vi "通信并与其他模块交互 (子VI).vi"() -> ()   [LabVIEW 2016, in "质控单元.lvlib"]
uses:
  <vilib>/Plasmionique/MB Master/MB_Master_TCP/MB_Master_TCP.lvclass
  D:/Program Files (x86)/National Instruments/LabVIEW 2016/vi.lib/Plasmionique/MB Master/MB_Master/MB_Master.lvclass
  <vilib>/Plasmionique/MB Master/MB_Master/MB_Master.lvclass
  <vilib>/Plasmionique/MB Master/MB Master.lvlib
  <vilib>/Utility/config.llb/NI_LVConfig.lvlib
panel:
  out "CODCr测量状态":u16[](array[numeric])
  out "CODMn测量状态":u16[](array[numeric])
  out "总氮测量状态":u16[](array[numeric])
  out "总磷测量状态":u16[](array[numeric])
  out "氨氮测量状态":u16[](array[numeric])
  out "通讯状态":bool
  out "待处理插入数量":i32
  out "元素":cluster{"命令":string}[](array[cluster])
  out "队列中元素数量":i32
  in  "starting address 6":u16
  in  "values 6":u16[](array[numeric])
  in  "starting address 5":u16
  in  "values 5":u16[](array[numeric])
  in  "starting address 4":u16
  in  "values 4":u16[](array[numeric])
  in  "starting address 3":u16
  in  "values 3":u16[](array[numeric])
  in  "starting address 2":u16
  in  "values 2":u16[](array[numeric])
  in  "values":u16[](array[numeric])
  in  "starting address":u16
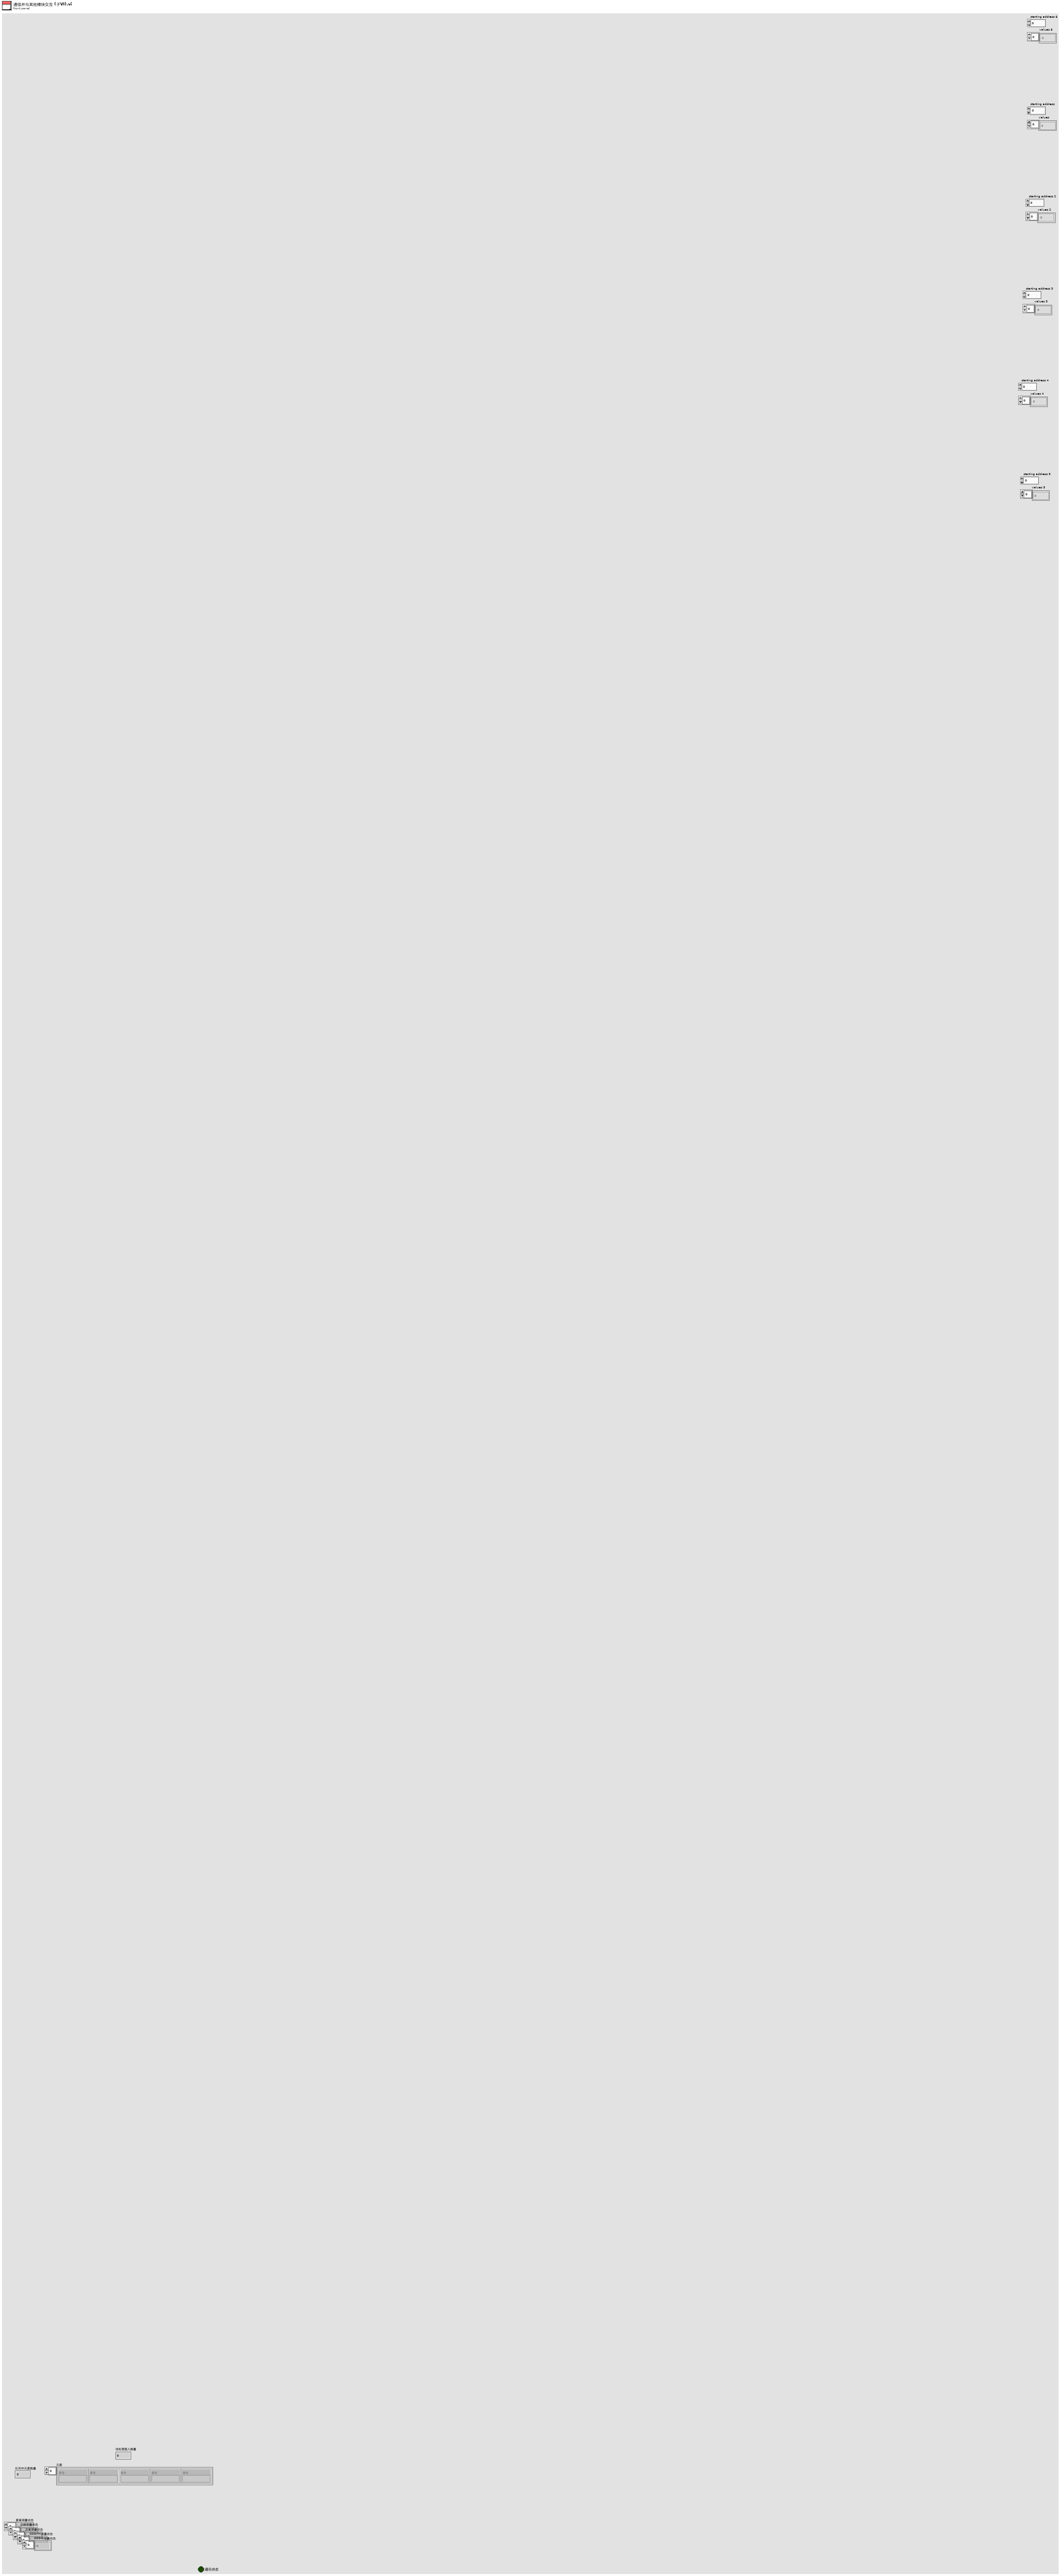
[diagram p1: front panel]
types:
  T1 = typedef "NI_LVConfig.lvlib/Config Data RefNum.ctl" = refnum<k1>
  T2 = cluster{"因子编码":u32, "单位":u16, "标样参考值":sgl, "水样数据时间":timestamp, "水样实测值":sgl, "水样数据标识":string, "标样数据时间":timestamp, "标样实测值":sgl, "标样数据标识":string, "空白数据时间":timestamp, "空白实测值":sgl, "空白数据标识":string, "零点核查数据时间":timestamp, "零点核查实测值":sgl, "零点核查数据标识":string, "跨度核查数据时间":timestamp, "跨度核查实测值":sgl, "跨度核查数据标识":string, "加标回收数据时间":timestamp, "加标回收实测值":sgl, "加标回收数据标识":string, "平行样数据时间":timestamp, "平行样实测值":sgl, "平行样数据标识":string}
  T3 = cluster{"系统时间":timestamp, "工作状态":enum16{"空闲", "水样测试", "标样核查", "零点核查", "跨度核查", "空白测试", "平行样测试", "加标回收", "空白校准", "标样校准", "初始化（清洗）"}, "测量模式":enum16{"待机", "连续模式", "周期模式", "定点模式", "受控模式", "手动模式"}, "告警代码":enum16{"无告警", "缺试剂告警", "缺水样告警", "缺蒸馏水告警", "缺标液告警", "仪表漏液告警", "标定异常告警", "超量程告警", "加热异常", "低试剂预警", "超上限告警", "超下限告警", "仪表内部其他异常", "滴定异常告警", "电极异常告警", "量程切换告警", "参数设置告警", "PH电极电位异常", "电导率电极异常", "浊度光度异常", "溶解氧电极异常", "溶解氧光强异常", "温度异常告警", "PH异常告警", "溶解氧异常告警", "电导率异常告警", "浊度异常告警", "叶绿素异常告警", "藻密度异常告警", "蓝绿藻异常告警", "ORP异常告警", "氨氮异常告警", "清洁刷异常告警", "SD卡异常告警", "蓝牙异常告警", "Wifi异常告警", "流程异常告警"}, "故障代码":enum16{"无故障", "电机故障", "温度故障", "通讯故障", "滴定故障"}, "日志代码":u16, "软件版本":u16, "F0":sgl, "F1":sgl, "F2":sgl, "F3":sgl, "T":sgl, "H":sgl, "id":u16, "flowid":u16, "量程":u16, "总磷控温温度1":sgl, "营养盐控温温度2":sgl, "ADC":sgl}
  T4 = cluster{"Registers[0]":u16, "Registers[1]":u16, "Registers[2]":u16, "Registers[3]":u16, "Registers[4]":u16, "Registers[5]":u16, "Registers[6]":u16, "Registers[7]":u16, "Registers[8]":u16, "Registers[9]":u16, "Registers[10]":u16, "Registers[11]":u16, "Registers[12]":u16, "Registers[13]":u16, "Registers[14]":u16, "Registers[15]":u16, "Registers[16]":u16, "Registers[17]":u16, "Registers[18]":u16, "Registers[19]":u16, "Registers[20]":u16, "Registers[21]":u16, "Registers[22]":u16, "Registers[23]":u16, "Registers[24]":u16, "Registers[25]":u16, "Registers[26]":u16, "Registers[27]":u16, "Registers[28]":u16, "Registers[29]":u16, "Registers[30]":u16, "Registers[31]":u16, "Registers[32]":u16, "Registers[33]":u16, "Registers[34]":u16, "Registers[35]":u16, "Registers[36]":u16, "Registers[37]":u16, "Registers[38]":u16, "Registers[39]":u16, "Registers[40]":u16, "Registers[41]":u16, "Registers[42]":u16, "Registers[43]":u16, "Registers[44]":u16, "Registers[45]":u16, "Registers[46]":u16, "Registers[47]":u16, "Registers[48]":u16, "Registers[49]":u16, "Registers[50]":u16, "Registers[51]":u16, "Registers[52]":u16, "Registers[53]":u16, "Registers[54]":u16, "Registers[55]":u16, "Registers[56]":u16}
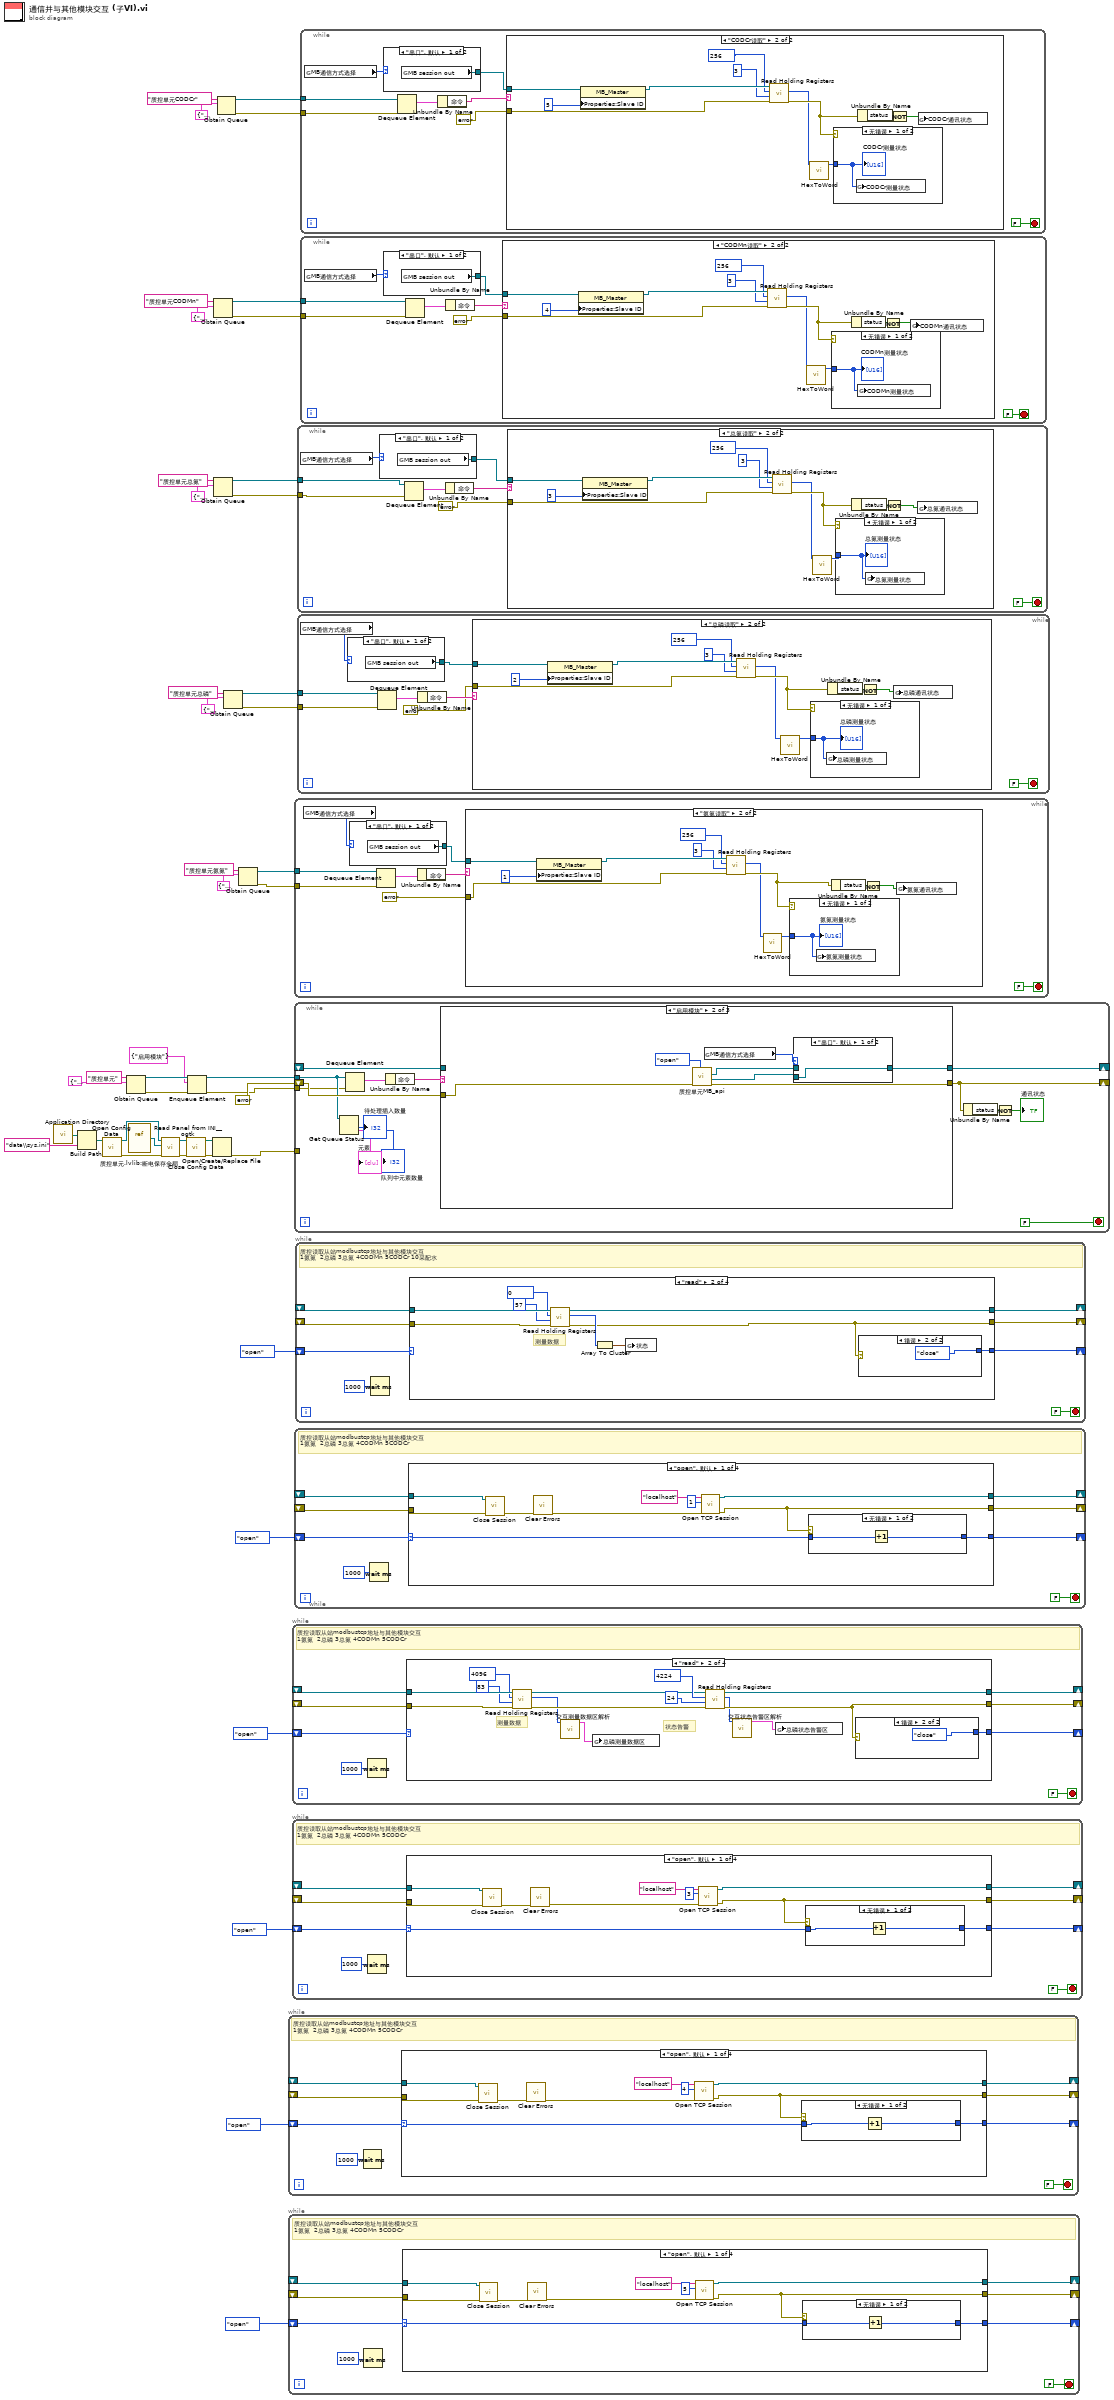
[diagram p0: block diagram]
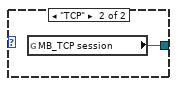
[diagram p2: hidden frame]
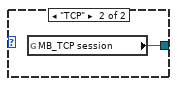
[diagram p5: hidden frame]
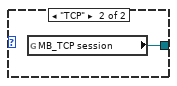
[diagram p8: hidden frame]
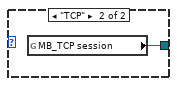
[diagram p11: hidden frame]
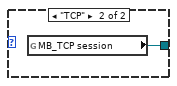
[diagram p14: hidden frame]
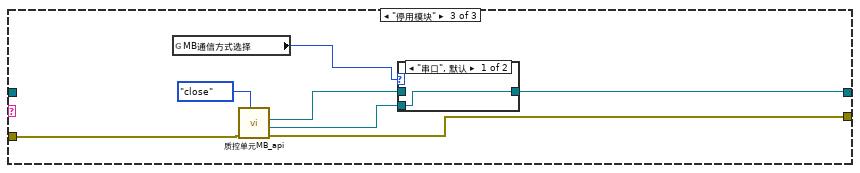
[diagram p19: hidden frame]
diagram:
  n1 = call <vilib>:"Application Directory.vi"() -> ("Application Directory"=w33:path)
  n2 = Build Path(base path=w33, name or relative path="data\\sys.ini" ("名称或相对路径")) -> (appended path=w31:path)
  n3 = call <vilib>:"Open Config Data.vi"("configuration file path"=w31) -> ("error out"=w27:errorcluster, "refnum"=w30:T1)  [unwired: 8 in, 1 out]
  n4 = Obtain Queue(name (unnamed)="质控单元" ("名称（未命名）"), element data type=cluster{"命令":string} {"命令"="启用模块"} ("元素")) -> (queue out=w36:refnum<queue>, error out=w35:errorcluster)  [unwired: 3 in, 1 out]
  n5 = vi-ref "质控单元.lvlib:断电保存全局.vi"() -> (w29:refnum<vi>)
  n6 = call <userlib>:"Read Panel from INI__ogtk.vi"("error in (no error)"=w27, "VI ref"=w29, "refnum"=w30) -> ("error out"=w26:errorcluster, "refnum out"=w28:T1)  [unwired: 7 in]
  n7 = call <vilib>:"Close Config Data.vi"("error in (no error)"=w26, "refnum"=w28) -> ("error out"=w25:errorcluster, "file path"=w24:path)  [unwired: 8 in]
  n8 = Enqueue Element(queue=w36, element=cluster{"命令":string} {"命令"="启用模块"} ("元素"), error in (no error)=w35) -> (queue out=w23:refnum<queue>, error out=w22:errorcluster)  [unwired: 1 in, 1 out]
  n9 = Open/Create/Replace File(file path (use dialog)=w24, error in=w25) -> (error out=w1:errorcluster)  [unwired: 4 in, 2 out]
  n10 = Obtain Queue(name (unnamed)="质控单元CODMn" ("名称（未命名）"), element data type=cluster{"命令":string} {"命令"="启用模块"} ("元素")) -> (queue out=w5:refnum<queue>, error out=w4:errorcluster)  [unwired: 3 in, 1 out]
  n11 = Obtain Queue(name (unnamed)="质控单元总氮" ("名称（未命名）"), element data type=cluster{"命令":string} {"命令"="启用模块"} ("元素")) -> (queue out=w7:refnum<queue>, error out=w6:errorcluster)  [unwired: 3 in, 1 out]
  n12 = Obtain Queue(name (unnamed)="质控单元CODCr" ("名称（未命名）"), element data type=cluster{"命令":string} {"命令"="启用模块"} ("元素")) -> (queue out=w3:refnum<queue>, error out=w2:errorcluster)  [unwired: 3 in, 1 out]
  n13 = Obtain Queue(name (unnamed)="质控单元总磷" ("名称（未命名）"), element data type=cluster{"命令":string} {"命令"="启用模块"} ("元素")) -> (queue out=w9:refnum<queue>, error out=w8:errorcluster)  [unwired: 3 in, 1 out]
  n14 = Obtain Queue(name (unnamed)="质控单元氨氮" ("名称（未命名）"), element data type=cluster{"命令":string} {"命令"="启用模块"} ("元素")) -> (queue out=w11:refnum<queue>, error out=w10:errorcluster)  [unwired: 3 in, 1 out]
  n15 = while {
    shift-right: [w51] -> _
    shift-left: _ -> [w53]
    shift-right: [w50] -> _
    shift-left: _ -> [w52]
    shift-right: [w47] -> _
    shift-left: enum16{"open", "read", "write", "close"}."open" -> [w48]
    stop <- FALSE stop-if-true
    # "质控读取从站modbustcp地址与其他模块交互\n1氨氮  2总磷 3总氮 4CODMn 5CODCr"
    n16 = Wait (ms)(milliseconds to wait=u32 1000 ("等待时间（毫秒）")) -> ()  [unwired: 1 out]
    n17 = case shown="\"open\", 默认" w48 {
      selector: w48 -> [w55 _ _ _]
      tunnel: w53 -> [w60 w91 w99 w107]
      tunnel: w52 -> [w59 w88 w98 w106]
      tunnel: [w61 w86 w97 w107] -> w51
      tunnel: [w56 w85 w96 w104] -> w50
      tunnel: [w54 w87 w100 enum16{"open", "read", "write", "close"}."open"] -> w47
      frame "open", Default {
        n18 = call-dynamic "Close Session.vi"("error in (no error)"=w59, "MB session in"=w60) -> ("error out"=w58:errorcluster)  [unwired: 9 in]
        n19 = call <vilib>:"Clear Errors.vi"("error in (no error)"=w58) -> ("error out"=w57:errorcluster)  [unwired: 5 in, 1 out]
        n20 = call <vilib>:"Open TCP Session.vi"("error in (no error)"=w57, "Port (502)"=u16 4, "IP Address"="localhost") -> ("error out"=w56:errorcluster, "MB_TCP session"=w61:refnum<class "MB_Master_TCP.lvclass">)  [unwired: 7 in]
        n21 = case shown="无错误" w56 {
          tunnel: w55 -> [w65 w66]
          tunnel: [w64 w66] -> w54
          frame No Error {
            n22 = Increment(x=w65) -> (x+1=w64:enum16{"open", "read", "write", "close"})
          }
          frame Error {
          }
        }
      }
      frame "read" {
        # "测量数据"
        n23 = call <vilib>:"Read Holding Registers.vi"("error in (no error)"=w88, "quantity"=u16 30, "starting address"=u16 0, "MB session in"=w91) -> ("error out"=w85:errorcluster, "Registers"=w84:u16[], "MB session out"=w86:refnum<class "MB_Master.lvclass">)  [unwired: 5 in]
        n24 = Index Array(array=w84) -> (element #1=w83:u16, element #2=w82:u16, element #3=w81:u16, element #4=w77:u16, element #5=w76:u16, element #6=w75:u16, element #7=w74:u16, element #8=w72:u16, element #9=w71:u16, element #10=w70:u16)  [unwired: 10 in]
        n25 = Build Array(w82, w81) -> (w80:u16[])
        n26 = Build Array(w76, w75, w74, w72, w71, w70) -> (w73:u16[])
        n27 = call "HexToDate.vi"("数组"=w73) -> ("DATE"=w69:timestamp[])  [unwired: 10 in]
        n28 = call "HexToCDABFloat.vi"("数组"=w80) -> ("FLOAT"=w79:sgl[])  [unwired: 10 in]
        n29 = Index Array(array=w69) -> (element #1=w68:timestamp, element #2=w67:timestamp)  [unwired: 2 in]
        n30 = Index Array(array=w79) -> (element=w78:sgl)  [unwired: 1 in]
        n31 = global write "与CODMn交互全局.vi" "COD浓度（mg/L)"(w78) -> ()
        n32 = global write "与CODMn交互全局.vi" "加标回收启动时间"(w68) -> ()
        n33 = global write "与CODMn交互全局.vi" "CODMn工作状态"(w83) -> ()
        n34 = global write "与CODMn交互全局.vi" "水样启动时间"(w67) -> ()
        n35 = global write "与CODMn交互全局.vi" "多列列表框"(w77) -> ()
        n36 = case shown="错误" w85 {
          tunnel: [enum16{"open", "read", "write", "close"}."read" enum16{"open", "read", "write", "close"}."close"] -> w87
          frame No Error {
          }
          frame Error {
          }
        }
      }
      frame "write" {
        n37 = call <vilib>:"Write Multiple Registers.vi"("error in (no error)"=w98, "values"="values 4", "starting address"="starting address 4", "MB session in"=w99) -> ("error out"=w96:errorcluster, "MB session out"=w97:refnum<class "MB_Master.lvclass">)  [unwired: 6 in]
        n38 = case shown="错误" w96 {
          tunnel: [enum16{"open", "read", "write", "close"}."read" enum16{"open", "read", "write", "close"}."close"] -> w100
          frame No Error {
          }
          frame Error {
          }
        }
      }
      frame "close" {
        n39 = call-dynamic "Close Session.vi"("error in (no error)"=w106, "MB session in"=w107) -> ("error out"=w105:errorcluster)  [unwired: 9 in]
        n40 = call <vilib>:"Clear Errors.vi"("error in (no error)"=w105) -> ("error out"=w104:errorcluster)  [unwired: 5 in, 1 out]
      }
    }
  }
  n41 = while {
    shift-right: [w113] -> _
    shift-left: _ -> [w115]
    shift-right: [w112] -> _
    shift-left: _ -> [w114]
    shift-right: [w109] -> _
    shift-left: enum16{"open", "read", "write", "close"}."open" -> [w110]
    stop <- FALSE stop-if-true
    # "质控读取从站modbustcp地址与其他模块交互\n1氨氮  2总磷 3总氮 4CODMn 5CODCr"
    n42 = Wait (ms)(milliseconds to wait=u32 1000 ("等待时间（毫秒）")) -> ()  [unwired: 1 out]
    n43 = case shown="\"open\", 默认" w110 {
      selector: w110 -> [w117 _ _ _]
      tunnel: w115 -> [w122 w143 w151 w159]
      tunnel: w114 -> [w121 w140 w150 w158]
      tunnel: [w123 w134 w149 w159] -> w113
      tunnel: [w118 w133 w148 w156] -> w112
      tunnel: [w116 w139 w152 enum16{"open", "read", "write", "close"}."open"] -> w109
      frame "open", Default {
        n44 = call-dynamic "Close Session.vi"("error in (no error)"=w121, "MB session in"=w122) -> ("error out"=w120:errorcluster)  [unwired: 9 in]
        n45 = call <vilib>:"Clear Errors.vi"("error in (no error)"=w120) -> ("error out"=w119:errorcluster)  [unwired: 5 in, 1 out]
        n46 = call <vilib>:"Open TCP Session.vi"("error in (no error)"=w119, "Port (502)"=u16 5, "IP Address"="localhost") -> ("error out"=w118:errorcluster, "MB_TCP session"=w123:refnum<class "MB_Master_TCP.lvclass">)  [unwired: 7 in]
        n47 = case shown="无错误" w118 {
          tunnel: w117 -> [w127 w128]
          tunnel: [w126 w128] -> w116
          frame No Error {
            n48 = Increment(x=w127) -> (x+1=w126:enum16{"open", "read", "write", "close"})
          }
          frame Error {
          }
        }
      }
      frame "read" {
        # "状态告警"
        # "测量数据"
        n49 = call <vilib>:"Read Holding Registers.vi"("error in (no error)"=w140, "quantity"=u16 83, "starting address"=u16 4096, "MB session in"=w143) -> ("error out"=w135:errorcluster, "Registers"=w132:u16[], "MB session out"=w136:refnum<class "MB_Master.lvclass">)  [unwired: 5 in]
        n50 = call "交互测量数据区解析.vi"("数组"=w132) -> ("测量数据区"=w130:T2)  [unwired: 10 in]
        n51 = global write "与CODCr交互全局.vi" "CODCr测量数据区"(w130) -> ()
        n52 = call <vilib>:"Read Holding Registers.vi"("error in (no error)"=w135, "quantity"=u16 24, "starting address"=u16 4224, "MB session in"=w136) -> ("error out"=w133:errorcluster, "Registers"=w131:u16[], "MB session out"=w134:refnum<class "MB_Master.lvclass">)  [unwired: 5 in]
        n53 = call "交互状态告警区解析.vi"("数组"=w131) -> ("状态告警区"=w129:T3)  [unwired: 10 in]
        n54 = global write "与CODCr交互全局.vi" "CODCr状态告警区"(w129) -> ()
        n55 = case shown="错误" w133 {
          tunnel: [enum16{"open", "read", "write", "close"}."read" enum16{"open", "read", "write", "close"}."close"] -> w139
          frame No Error {
          }
          frame Error {
          }
        }
      }
      frame "write" {
        n56 = call <vilib>:"Write Multiple Registers.vi"("error in (no error)"=w150, "values"="values 5", "starting address"="starting address 5", "MB session in"=w151) -> ("error out"=w148:errorcluster, "MB session out"=w149:refnum<class "MB_Master.lvclass">)  [unwired: 6 in]
        n57 = case shown="错误" w148 {
          tunnel: [enum16{"open", "read", "write", "close"}."read" enum16{"open", "read", "write", "close"}."close"] -> w152
          frame No Error {
          }
          frame Error {
          }
        }
      }
      frame "close" {
        n58 = call-dynamic "Close Session.vi"("error in (no error)"=w158, "MB session in"=w159) -> ("error out"=w157:errorcluster)  [unwired: 9 in]
        n59 = call <vilib>:"Clear Errors.vi"("error in (no error)"=w157) -> ("error out"=w156:errorcluster)  [unwired: 5 in, 1 out]
      }
    }
  }
  n60 = while {
    shift-right: [w165] -> _
    shift-left: _ -> [w167]
    shift-right: [w164] -> _
    shift-left: _ -> [w166]
    shift-right: [w161] -> _
    shift-left: enum16{"open", "read", "write", "close"}."open" -> [w162]
    stop <- FALSE stop-if-true
    # "质控读取从站modbustcp地址与其他模块交互\n1氨氮  2总磷 3总氮 4CODMn 5CODCr"
    n61 = Wait (ms)(milliseconds to wait=u32 1000 ("等待时间（毫秒）")) -> ()  [unwired: 1 out]
    n62 = case shown="\"read\"" w162 {
      selector: w162 -> [w169 _ _ _]
      tunnel: w167 -> [w174 w195 w203 w211]
      tunnel: w166 -> [w173 w192 w202 w210]
      tunnel: [w175 w186 w201 w211] -> w165
      tunnel: [w170 w185 w200 w208] -> w164
      tunnel: [w168 w191 w204 enum16{"open", "read", "write", "close"}."open"] -> w161
      frame "open", Default {
        n63 = call-dynamic "Close Session.vi"("error in (no error)"=w173, "MB session in"=w174) -> ("error out"=w172:errorcluster)  [unwired: 9 in]
        n64 = call <vilib>:"Clear Errors.vi"("error in (no error)"=w172) -> ("error out"=w171:errorcluster)  [unwired: 5 in, 1 out]
        n65 = call <vilib>:"Open TCP Session.vi"("error in (no error)"=w171, "Port (502)"=u16 2, "IP Address"="localhost") -> ("error out"=w170:errorcluster, "MB_TCP session"=w175:refnum<class "MB_Master_TCP.lvclass">)  [unwired: 7 in]
        n66 = case shown="无错误" w170 {
          tunnel: w169 -> [w179 w180]
          tunnel: [w178 w180] -> w168
          frame No Error {
            n67 = Increment(x=w179) -> (x+1=w178:enum16{"open", "read", "write", "close"})
          }
          frame Error {
          }
        }
      }
      frame "read" {
        # "状态告警"
        # "测量数据"
        n68 = call <vilib>:"Read Holding Registers.vi"("error in (no error)"=w192, "quantity"=u16 83, "starting address"=u16 4096, "MB session in"=w195) -> ("error out"=w187:errorcluster, "Registers"=w184:u16[], "MB session out"=w188:refnum<class "MB_Master.lvclass">)  [unwired: 5 in]
        n69 = call "交互测量数据区解析.vi"("数组"=w184) -> ("测量数据区"=w182:T2)  [unwired: 10 in]
        n70 = global write "与总磷交互全局.vi" "总磷测量数据区"(w182) -> ()
        n71 = call <vilib>:"Read Holding Registers.vi"("error in (no error)"=w187, "quantity"=u16 24, "starting address"=u16 4224, "MB session in"=w188) -> ("error out"=w185:errorcluster, "Registers"=w183:u16[], "MB session out"=w186:refnum<class "MB_Master.lvclass">)  [unwired: 5 in]
        n72 = call "交互状态告警区解析.vi"("数组"=w183) -> ("状态告警区"=w181:T3)  [unwired: 10 in]
        n73 = global write "与总磷交互全局.vi" "总磷状态告警区"(w181) -> ()
        n74 = case shown="错误" w185 {
          tunnel: [enum16{"open", "read", "write", "close"}."read" enum16{"open", "read", "write", "close"}."close"] -> w191
          frame No Error {
          }
          frame Error {
          }
        }
      }
      frame "write" {
        n75 = call <vilib>:"Write Multiple Registers.vi"("error in (no error)"=w202, "values"="values 2", "starting address"="starting address 2", "MB session in"=w203) -> ("error out"=w200:errorcluster, "MB session out"=w201:refnum<class "MB_Master.lvclass">)  [unwired: 6 in]
        n76 = case shown="错误" w200 {
          tunnel: [enum16{"open", "read", "write", "close"}."read" enum16{"open", "read", "write", "close"}."close"] -> w204
          frame No Error {
          }
          frame Error {
          }
        }
      }
      frame "close" {
        n77 = call-dynamic "Close Session.vi"("error in (no error)"=w210, "MB session in"=w211) -> ("error out"=w209:errorcluster)  [unwired: 9 in]
        n78 = call <vilib>:"Clear Errors.vi"("error in (no error)"=w209) -> ("error out"=w208:errorcluster)  [unwired: 5 in, 1 out]
      }
    }
  }
  n79 = while {
    shift-right: [w217] -> _
    shift-left: _ -> [w219]
    shift-right: [w216] -> _
    shift-left: _ -> [w218]
    shift-right: [w213] -> _
    shift-left: enum16{"open", "read", "write", "close"}."open" -> [w214]
    stop <- FALSE stop-if-true
    # "质控读取从站modbustcp地址与其他模块交互\n1氨氮  2总磷 3总氮 4CODMn 5CODCr"
    n80 = Wait (ms)(milliseconds to wait=u32 1000 ("等待时间（毫秒）")) -> ()  [unwired: 1 out]
    n81 = case shown="\"open\", 默认" w214 {
      selector: w214 -> [w221 _ _ _]
      tunnel: w219 -> [w226 w247 w255 w263]
      tunnel: w218 -> [w225 w244 w254 w262]
      tunnel: [w227 w238 w253 w263] -> w217
      tunnel: [w222 w237 w252 w260] -> w216
      tunnel: [w220 w243 w256 enum16{"open", "read", "write", "close"}."open"] -> w213
      frame "open", Default {
        n82 = call-dynamic "Close Session.vi"("error in (no error)"=w225, "MB session in"=w226) -> ("error out"=w224:errorcluster)  [unwired: 9 in]
        n83 = call <vilib>:"Clear Errors.vi"("error in (no error)"=w224) -> ("error out"=w223:errorcluster)  [unwired: 5 in, 1 out]
        n84 = call <vilib>:"Open TCP Session.vi"("error in (no error)"=w223, "Port (502)"=u16 3, "IP Address"="localhost") -> ("error out"=w222:errorcluster, "MB_TCP session"=w227:refnum<class "MB_Master_TCP.lvclass">)  [unwired: 7 in]
        n85 = case shown="无错误" w222 {
          tunnel: w221 -> [w231 w232]
          tunnel: [w230 w232] -> w220
          frame No Error {
            n86 = Increment(x=w231) -> (x+1=w230:enum16{"open", "read", "write", "close"})
          }
          frame Error {
          }
        }
      }
      frame "read" {
        # "状态告警"
        # "测量数据"
        n87 = call <vilib>:"Read Holding Registers.vi"("error in (no error)"=w244, "quantity"=u16 83, "starting address"=u16 4096, "MB session in"=w247) -> ("error out"=w239:errorcluster, "Registers"=w236:u16[], "MB session out"=w240:refnum<class "MB_Master.lvclass">)  [unwired: 5 in]
        n88 = call "交互测量数据区解析.vi"("数组"=w236) -> ("测量数据区"=w234:T2)  [unwired: 10 in]
        n89 = global write "与总氮交互全局.vi" "总氮测量数据区"(w234) -> ()
        n90 = call <vilib>:"Read Holding Registers.vi"("error in (no error)"=w239, "quantity"=u16 24, "starting address"=u16 4224, "MB session in"=w240) -> ("error out"=w237:errorcluster, "Registers"=w235:u16[], "MB session out"=w238:refnum<class "MB_Master.lvclass">)  [unwired: 5 in]
        n91 = call "交互状态告警区解析.vi"("数组"=w235) -> ("状态告警区"=w233:T3)  [unwired: 10 in]
        n92 = global write "与总氮交互全局.vi" "总氮状态告警区"(w233) -> ()
        n93 = case shown="错误" w237 {
          tunnel: [enum16{"open", "read", "write", "close"}."read" enum16{"open", "read", "write", "close"}."close"] -> w243
          frame No Error {
          }
          frame Error {
          }
        }
      }
      frame "write" {
        n94 = call <vilib>:"Write Multiple Registers.vi"("error in (no error)"=w254, "values"="values 3", "starting address"="starting address 3", "MB session in"=w255) -> ("error out"=w252:errorcluster, "MB session out"=w253:refnum<class "MB_Master.lvclass">)  [unwired: 6 in]
        n95 = case shown="错误" w252 {
          tunnel: [enum16{"open", "read", "write", "close"}."read" enum16{"open", "read", "write", "close"}."close"] -> w256
          frame No Error {
          }
          frame Error {
          }
        }
      }
      frame "close" {
        n96 = call-dynamic "Close Session.vi"("error in (no error)"=w262, "MB session in"=w263) -> ("error out"=w261:errorcluster)  [unwired: 9 in]
        n97 = call <vilib>:"Clear Errors.vi"("error in (no error)"=w261) -> ("error out"=w260:errorcluster)  [unwired: 5 in, 1 out]
      }
    }
  }
  n98 = while {
    tunnel: w23 -> [w276]
    tunnel: w22 -> [w275]
    shift-right: [w267] -> _
    shift-left: _ -> [w266]
    tunnel: w1 -> [_]
    shift-right: [w265] -> _
    shift-left: errorcluster {"status"=FALSE, "code"=0, "source"=""} ("error out") -> [w277]
    stop <- FALSE stop-if-true
    n99 = Get Queue Status(queue=w276) -> (# pending insert=→"待处理插入数量":i32, # elements in queue=→"队列中元素数量":i32, elements=→"元素":cluster{"命令":string}[])  [unwired: 2 in, 5 out]
    n100 = Dequeue Element(queue=w276, error in (no error)=w275) -> (element=w274:cluster{"命令":string})  [unwired: 1 in, 3 out]
    n101 = Unbundle By Name(w274) -> ("命令"=w273:string)
    n102 = case shown="\"启用模块\"" w273 {
      tunnel: [w279 w281 w291] -> w267
      tunnel: [w278 w286 w293] -> w265
      tunnel: w266 -> [w279 _ _]
      tunnel: w277 -> [w278 w284 w294]
      frame Default {
      }
      frame "启用模块" {
        n103 = call "质控单元MB_api.vi"("STEP"=enum16{"open", "read", "write", "close"}."open", "Error in"=w284) -> ("error out"=w286:errorcluster, "MB session out"=w282:refnum<class "MB_Master.lvclass">, "MB_TCP session"=w283:refnum<class "MB_Master_TCP.lvclass">)  [unwired: 6 in, 1 out]
        n104 = global read "断电保存全局.vi" "MB通信方式选择"() -> (w280:enum16{"串口", "TCP"})
        n105 = case shown="\"串口\", 默认" w280 {
          tunnel: w283 -> [_ w288]
          tunnel: w282 -> [w287 _]
          tunnel: [w287 w288] -> w281
          frame "串口", Default {
          }
          frame "TCP" {
          }
        }
      }
      frame "停用模块" {
        n106 = global read "断电保存全局.vi" "MB通信方式选择"() -> (w289:enum16{"串口", "TCP"})
        n107 = call "质控单元MB_api.vi"("STEP"=enum16{"open", "read", "write", "close"}."close", "Error in"=w294) -> ("error out"=w293:errorcluster, "MB session out"=w292:refnum<class "MB_Master.lvclass">, "MB_TCP session"=w290:refnum<class "MB_Master_TCP.lvclass">)  [unwired: 6 in, 1 out]
        n108 = case shown="\"串口\", 默认" w289 {
          tunnel: w290 -> [_ w297]
          tunnel: w292 -> [w296 _]
          tunnel: [w296 w297] -> w291
          frame "串口", Default {
          }
          frame "TCP" {
          }
        }
      }
    }
    n109 = Unbundle By Name(w265) -> ("status"=w272:bool)
    n110 = Not(x=w272) -> (.not. x?=→"通讯状态":bool)
  }
  n111 = while {
    tunnel: w11 -> [w305]
    tunnel: w10 -> [w304]
    stop <- FALSE stop-if-true
    n112 = global read "断电保存全局.vi" "MB通信方式选择"() -> (w301:enum16{"串口", "TCP"})
    n113 = case shown="\"串口\", 默认" w301 {
      tunnel: [w306 w307] -> w300
      frame "串口", Default {
        n114 = global read "断电保存全局.vi" "MB session out"() -> (w306:refnum<class "MB_Master.lvclass">)
      }
      frame "TCP" {
        n115 = global read "断电保存全局.vi" "MB_TCP session"() -> (w307:refnum<class "MB_Master_TCP.lvclass">)
      }
    }
    n116 = Dequeue Element(queue=w305, error in (no error)=w304) -> (element=w303:cluster{"命令":string})  [unwired: 1 in, 3 out]
    n117 = Unbundle By Name(w303) -> ("命令"=w302:string)
    n118 = case shown="\"氨氮读取\"" w302 {
      tunnel: errorcluster {"status"=FALSE, "code"=0, "source"=""} ("error out") -> [_ w311]
      tunnel: w300 -> [_ w310]
      frame "假", Default {
      }
      frame "氨氮读取" {
        n119 = property class="MB_Master"(reference=w310, "Properties:Slave ID"=u8 1 ("Slave ID")) -> (reference out=w315:refnum<class "MB_Master.lvclass">)  [unwired: 1 in, 1 out]
        n120 = call <vilib>:"Read Holding Registers.vi"("error in (no error)"=w311, "quantity"=u16 3 ("number of holding registers"), "starting address"=u16 256, "MB session in"=w315) -> ("error out"=w317:errorcluster, "Registers"=w309:u16[])  [unwired: 5 in, 1 out]
        n121 = call "HexToWord.vi"("数组"=w309) -> ("WORD"=w308:u16[])  [unwired: 10 in]
        n122 = case shown="无错误" w317 {
          tunnel: w308 -> [w319 _]
          frame No Error {
            n123 = global write "质控内部交互全局.vi" "氨氮测量状态"(w319) -> ()
            "氨氮测量状态" <- w319
          }
          frame Error {
          }
        }
        n124 = Unbundle By Name(w317) -> ("status"=w316:bool)
        n125 = Not(x=w316) -> (.not. x?=w318:bool)
        n126 = global write "质控内部交互全局.vi" "氨氮通讯状态"(w318) -> ()
      }
    }
  }
  n127 = while {
    shift-right: [w325] -> _
    shift-left: _ -> [w327]
    shift-right: [w324] -> _
    shift-left: _ -> [w326]
    shift-right: [w321] -> _
    shift-left: enum16{"open", "read", "write", "close"}."open" -> [w322]
    stop <- FALSE stop-if-true
    # "质控读取从站modbustcp地址与其他模块交互\n1氨氮  2总磷 3总氮 4CODMn 5CODCr"
    n128 = Wait (ms)(milliseconds to wait=u32 1000 ("等待时间（毫秒）")) -> ()  [unwired: 1 out]
    n129 = case shown="\"open\", 默认" w322 {
      selector: w322 -> [w329 _ _ _]
      tunnel: w327 -> [w334 w355 w363 w371]
      tunnel: w326 -> [w333 w352 w362 w370]
      tunnel: [w335 w346 w361 w371] -> w325
      tunnel: [w330 w345 w360 w368] -> w324
      tunnel: [w328 w351 w364 enum16{"open", "read", "write", "close"}."open"] -> w321
      frame "open", Default {
        n130 = call-dynamic "Close Session.vi"("error in (no error)"=w333, "MB session in"=w334) -> ("error out"=w332:errorcluster)  [unwired: 9 in]
        n131 = call <vilib>:"Clear Errors.vi"("error in (no error)"=w332) -> ("error out"=w331:errorcluster)  [unwired: 5 in, 1 out]
        n132 = call <vilib>:"Open TCP Session.vi"("error in (no error)"=w331, "Port (502)"=u16 1, "IP Address"="localhost") -> ("error out"=w330:errorcluster, "MB_TCP session"=w335:refnum<class "MB_Master_TCP.lvclass">)  [unwired: 7 in]
        n133 = case shown="无错误" w330 {
          tunnel: w329 -> [w339 w340]
          tunnel: [w338 w340] -> w328
          frame No Error {
            n134 = Increment(x=w339) -> (x+1=w338:enum16{"open", "read", "write", "close"})
          }
          frame Error {
          }
        }
      }
      frame "read" {
        # "状态告警"
        # "测量数据"
        n135 = call <vilib>:"Read Holding Registers.vi"("error in (no error)"=w352, "quantity"=u16 83, "starting address"=u16 4096, "MB session in"=w355) -> ("error out"=w347:errorcluster, "Registers"=w344:u16[], "MB session out"=w348:refnum<class "MB_Master.lvclass">)  [unwired: 5 in]
        n136 = call "交互测量数据区解析.vi"("数组"=w344) -> ("测量数据区"=w343:T2)  [unwired: 10 in]
        n137 = global write "与氨氮交互全局.vi" "氨氮测量数据区"(w343) -> ()
        n138 = call <vilib>:"Read Holding Registers.vi"("error in (no error)"=w347, "quantity"=u16 24, "starting address"=u16 4224, "MB session in"=w348) -> ("error out"=w345:errorcluster, "Registers"=w342:u16[], "MB session out"=w346:refnum<class "MB_Master.lvclass">)  [unwired: 5 in]
        n139 = call "交互状态告警区解析.vi"("数组"=w342) -> ("状态告警区"=w341:T3)  [unwired: 10 in]
        n140 = global write "与氨氮交互全局.vi" "氨氮状态告警区"(w341) -> ()
        n141 = case shown="错误" w345 {
          tunnel: [enum16{"open", "read", "write", "close"}."read" enum16{"open", "read", "write", "close"}."close"] -> w351
          frame No Error {
          }
          frame Error {
          }
        }
      }
      frame "write" {
        n142 = call <vilib>:"Write Multiple Registers.vi"("error in (no error)"=w362, "values"="values", "starting address"="starting address", "MB session in"=w363) -> ("error out"=w360:errorcluster, "MB session out"=w361:refnum<class "MB_Master.lvclass">)  [unwired: 6 in]
        n143 = case shown="错误" w360 {
          tunnel: [enum16{"open", "read", "write", "close"}."read" enum16{"open", "read", "write", "close"}."close"] -> w364
          frame No Error {
          }
          frame Error {
          }
        }
      }
      frame "close" {
        n144 = call-dynamic "Close Session.vi"("error in (no error)"=w370, "MB session in"=w371) -> ("error out"=w369:errorcluster)  [unwired: 9 in]
        n145 = call <vilib>:"Clear Errors.vi"("error in (no error)"=w369) -> ("error out"=w368:errorcluster)  [unwired: 5 in, 1 out]
      }
    }
  }
  n146 = while {
    shift-right: [w377] -> _
    shift-left: _ -> [w379]
    shift-right: [w376] -> _
    shift-left: _ -> [w378]
    shift-right: [w373] -> _
    shift-left: enum16{"open", "read", "write", "close"}."open" -> [w374]
    stop <- FALSE stop-if-true
    # "质控读取从站modbustcp地址与其他模块交互\n1氨氮  2总磷 3总氮 4CODMn 5CODCr 10采配水"
    n147 = Wait (ms)(milliseconds to wait=u32 1000 ("等待时间（毫秒）")) -> ()  [unwired: 1 out]
    n148 = case shown="\"read\"" w374 {
      selector: w374 -> [w381 _ _ _]
      tunnel: w379 -> [w386 w401 w409 w417]
      tunnel: w378 -> [w385 w398 w408 w416]
      tunnel: [w387 w394 w407 w417] -> w377
      tunnel: [w382 w393 w406 w414] -> w376
      tunnel: [w380 w397 w410 enum16{"open", "read", "write", "close"}."open"] -> w373
      frame "open", Default {
        n149 = call-dynamic "Close Session.vi"("error in (no error)"=w385, "MB session in"=w386) -> ("error out"=w384:errorcluster)  [unwired: 9 in]
        n150 = call <vilib>:"Clear Errors.vi"("error in (no error)"=w384) -> ("error out"=w383:errorcluster)  [unwired: 5 in, 1 out]
        n151 = call <vilib>:"Open TCP Session.vi"("error in (no error)"=w383, "Port (502)"=u16 10, "IP Address"="localhost") -> ("error out"=w382:errorcluster, "MB_TCP session"=w387:refnum<class "MB_Master_TCP.lvclass">)  [unwired: 7 in]
        n152 = case shown="无错误" w382 {
          tunnel: w381 -> [w391 w392]
          tunnel: [w390 w392] -> w380
          frame No Error {
            n153 = Increment(x=w391) -> (x+1=w390:enum16{"open", "read", "write", "close"})
          }
          frame Error {
          }
        }
      }
      frame "read" {
        # "测量数据"
        n154 = call <vilib>:"Read Holding Registers.vi"("error in (no error)"=w398, "quantity"=u16 57, "starting address"=u16 0, "MB session in"=w401) -> ("error out"=w393:errorcluster, "Registers"=w396:u16[], "MB session out"=w394:refnum<class "MB_Master.lvclass">)  [unwired: 5 in]
        n155 = Array To Cluster(array=w396) -> (cluster=w395:T4)
        n156 = global write "与采配水交互全局.vi" "状态"(w395) -> ()
        n157 = case shown="错误" w393 {
          tunnel: [enum16{"open", "read", "write", "close"}."read" enum16{"open", "read", "write", "close"}."close"] -> w397
          frame No Error {
          }
          frame Error {
          }
        }
      }
      frame "write" {
        n158 = call <vilib>:"Write Multiple Registers.vi"("error in (no error)"=w408, "values"="values 6", "starting address"="starting address 6", "MB session in"=w409) -> ("error out"=w406:errorcluster, "MB session out"=w407:refnum<class "MB_Master.lvclass">)  [unwired: 6 in]
        n159 = case shown="错误" w406 {
          tunnel: [enum16{"open", "read", "write", "close"}."read" enum16{"open", "read", "write", "close"}."close"] -> w410
          frame No Error {
          }
          frame Error {
          }
        }
      }
      frame "close" {
        n160 = call-dynamic "Close Session.vi"("error in (no error)"=w416, "MB session in"=w417) -> ("error out"=w415:errorcluster)  [unwired: 9 in]
        n161 = call <vilib>:"Clear Errors.vi"("error in (no error)"=w415) -> ("error out"=w414:errorcluster)  [unwired: 5 in, 1 out]
      }
    }
  }
  n162 = while {
    tunnel: w7 -> [w425]
    tunnel: w6 -> [w424]
    stop <- FALSE stop-if-true
    n163 = global read "断电保存全局.vi" "MB通信方式选择"() -> (w421:enum16{"串口", "TCP"})
    n164 = case shown="\"串口\", 默认" w421 {
      tunnel: [w426 w427] -> w419
      frame "串口", Default {
        n165 = global read "断电保存全局.vi" "MB session out"() -> (w426:refnum<class "MB_Master.lvclass">)
      }
      frame "TCP" {
        n166 = global read "断电保存全局.vi" "MB_TCP session"() -> (w427:refnum<class "MB_Master_TCP.lvclass">)
      }
    }
    n167 = Dequeue Element(queue=w425, error in (no error)=w424) -> (element=w423:cluster{"命令":string})  [unwired: 1 in, 3 out]
    n168 = Unbundle By Name(w423) -> ("命令"=w422:string)
    n169 = case shown="\"总氮读取\"" w422 {
      tunnel: w419 -> [_ w432]
      tunnel: errorcluster {"status"=FALSE, "code"=0, "source"=""} ("error out") -> [_ w431]
      frame "假", Default {
      }
      frame "总氮读取" {
        n170 = property class="MB_Master"(reference=w432, "Properties:Slave ID"=u8 3 ("Slave ID")) -> (reference out=w435:refnum<class "MB_Master.lvclass">)  [unwired: 1 in, 1 out]
        n171 = call <vilib>:"Read Holding Registers.vi"("error in (no error)"=w431, "quantity"=u16 3 ("number of holding registers"), "starting address"=u16 256, "MB session in"=w435) -> ("error out"=w438:errorcluster, "Registers"=w430:u16[])  [unwired: 5 in, 1 out]
        n172 = call "HexToWord.vi"("数组"=w430) -> ("WORD"=w429:u16[])  [unwired: 10 in]
        n173 = case shown="无错误" w438 {
          tunnel: w429 -> [w439 _]
          frame No Error {
            n174 = global write "质控内部交互全局.vi" "总氮测量状态"(w439) -> ()
            "总氮测量状态" <- w439
          }
          frame Error {
          }
        }
        n175 = Unbundle By Name(w438) -> ("status"=w436:bool)
        n176 = Not(x=w436) -> (.not. x?=w437:bool)
        n177 = global write "质控内部交互全局.vi" "总氮通讯状态"(w437) -> ()
      }
    }
  }
  n178 = while {
    tunnel: w9 -> [w447]
    tunnel: w8 -> [w446]
    stop <- FALSE stop-if-true
    n179 = global read "断电保存全局.vi" "MB通信方式选择"() -> (w443:enum16{"串口", "TCP"})
    n180 = case shown="\"串口\", 默认" w443 {
      tunnel: [w448 w449] -> w442
      frame "串口", Default {
        n181 = global read "断电保存全局.vi" "MB session out"() -> (w448:refnum<class "MB_Master.lvclass">)
      }
      frame "TCP" {
        n182 = global read "断电保存全局.vi" "MB_TCP session"() -> (w449:refnum<class "MB_Master_TCP.lvclass">)
      }
    }
    n183 = Dequeue Element(queue=w447, error in (no error)=w446) -> (element=w445:cluster{"命令":string})  [unwired: 1 in, 3 out]
    n184 = Unbundle By Name(w445) -> ("命令"=w444:string)
    n185 = case shown="\"总磷读取\"" w444 {
      tunnel: w442 -> [_ w455]
      tunnel: errorcluster {"status"=FALSE, "code"=0, "source"=""} ("error out") -> [_ w454]
      frame "假", Default {
      }
      frame "总磷读取" {
        n186 = property class="MB_Master"(reference=w455, "Properties:Slave ID"=u8 2 ("Slave ID")) -> (reference out=w458:refnum<class "MB_Master.lvclass">)  [unwired: 1 in, 1 out]
        n187 = call <vilib>:"Read Holding Registers.vi"("error in (no error)"=w454, "quantity"=u16 3 ("number of holding registers"), "starting address"=u16 256, "MB session in"=w458) -> ("error out"=w453:errorcluster, "Registers"=w452:u16[])  [unwired: 5 in, 1 out]
        n188 = call "HexToWord.vi"("数组"=w452) -> ("WORD"=w451:u16[])  [unwired: 10 in]
        n189 = case shown="无错误" w453 {
          tunnel: w451 -> [w461 _]
          frame No Error {
            n190 = global write "质控内部交互全局.vi" "总磷测量状态"(w461) -> ()
            "总磷测量状态" <- w461
          }
          frame Error {
          }
        }
        n191 = Unbundle By Name(w453) -> ("status"=w459:bool)
        n192 = Not(x=w459) -> (.not. x?=w460:bool)
        n193 = global write "质控内部交互全局.vi" "总磷通讯状态"(w460) -> ()
      }
    }
  }
  n194 = while {
    tunnel: w3 -> [w469]
    tunnel: w2 -> [w468]
    stop <- FALSE stop-if-true
    n195 = global read "断电保存全局.vi" "MB通信方式选择"() -> (w465:enum16{"串口", "TCP"})
    n196 = case shown="\"串口\", 默认" w465 {
      tunnel: [w470 w471] -> w464
      frame "串口", Default {
        n197 = global read "断电保存全局.vi" "MB session out"() -> (w470:refnum<class "MB_Master.lvclass">)
      }
      frame "TCP" {
        n198 = global read "断电保存全局.vi" "MB_TCP session"() -> (w471:refnum<class "MB_Master_TCP.lvclass">)
      }
    }
    n199 = Dequeue Element(queue=w469, error in (no error)=w468) -> (element=w467:cluster{"命令":string})  [unwired: 1 in, 3 out]
    n200 = Unbundle By Name(w467) -> ("命令"=w466:string)
    n201 = case shown="\"CODCr读取\"" w466 {
      tunnel: w464 -> [_ w477]
      tunnel: errorcluster {"status"=FALSE, "code"=0, "source"=""} ("error out") -> [_ w476]
      frame "假", Default {
      }
      frame "CODCr读取" {
        n202 = property class="MB_Master"(reference=w477, "Properties:Slave ID"=u8 5 ("Slave ID")) -> (reference out=w481:refnum<class "MB_Master.lvclass">)  [unwired: 1 in, 1 out]
        n203 = call <vilib>:"Read Holding Registers.vi"("error in (no error)"=w476, "quantity"=u16 3 ("number of holding registers"), "starting address"=u16 256, "MB session in"=w481) -> ("error out"=w478:errorcluster, "Registers"=w475:u16[])  [unwired: 5 in, 1 out]
        n204 = call "HexToWord.vi"("数组"=w475) -> ("WORD"=w474:u16[])  [unwired: 10 in]
        n205 = case shown="无错误" w478 {
          tunnel: w474 -> [w483 _]
          frame No Error {
            n206 = global write "质控内部交互全局.vi" "CODCr测量状态"(w483) -> ()
            "CODCr测量状态" <- w483
          }
          frame Error {
          }
        }
        n207 = Unbundle By Name(w478) -> ("status"=w480:bool)
        n208 = Not(x=w480) -> (.not. x?=w479:bool)
        n209 = global write "质控内部交互全局.vi" "CODCr通讯状态"(w479) -> ()
      }
    }
  }
  n210 = while {
    tunnel: w5 -> [w491]
    tunnel: w4 -> [w490]
    stop <- FALSE stop-if-true
    n211 = global read "断电保存全局.vi" "MB通信方式选择"() -> (w487:enum16{"串口", "TCP"})
    n212 = case shown="\"串口\", 默认" w487 {
      tunnel: [w492 w493] -> w486
      frame "串口", Default {
        n213 = global read "断电保存全局.vi" "MB session out"() -> (w492:refnum<class "MB_Master.lvclass">)
      }
      frame "TCP" {
        n214 = global read "断电保存全局.vi" "MB_TCP session"() -> (w493:refnum<class "MB_Master_TCP.lvclass">)
      }
    }
    n215 = Dequeue Element(queue=w491, error in (no error)=w490) -> (element=w489:cluster{"命令":string})  [unwired: 1 in, 3 out]
    n216 = Unbundle By Name(w489) -> ("命令"=w488:string)
    n217 = case shown="\"CODMn读取\"" w488 {
      tunnel: w486 -> [_ w499]
      tunnel: errorcluster {"status"=FALSE, "code"=0, "source"=""} ("error out") -> [_ w498]
      frame "假", Default {
      }
      frame "CODMn读取" {
        n218 = property class="MB_Master"(reference=w499, "Properties:Slave ID"=u8 4 ("Slave ID")) -> (reference out=w503:refnum<class "MB_Master.lvclass">)  [unwired: 1 in, 1 out]
        n219 = call <vilib>:"Read Holding Registers.vi"("error in (no error)"=w498, "quantity"=u16 3 ("number of holding registers"), "starting address"=u16 256, "MB session in"=w503) -> ("error out"=w500:errorcluster, "Registers"=w497:u16[])  [unwired: 5 in, 1 out]
        n220 = call "HexToWord.vi"("数组"=w497) -> ("WORD"=w496:u16[])  [unwired: 10 in]
        n221 = case shown="无错误" w500 {
          tunnel: w496 -> [w505 _]
          frame No Error {
            n222 = global write "质控内部交互全局.vi" "CODMn测量状态"(w505) -> ()
            "CODMn测量状态" <- w505
          }
          frame Error {
          }
        }
        n223 = Unbundle By Name(w500) -> ("status"=w502:bool)
        n224 = Not(x=w502) -> (.not. x?=w501:bool)
        n225 = global write "质控内部交互全局.vi" "CODMn通讯状态"(w501) -> ()
      }
    }
  }
